vi "Set timebase horizontal scale.vi"(8 "error in (no error)":errorcluster, 9 "Horizontal timebase scale":dbl caption="Timebase horizontal scale", 11 "IVI Refnum in":refnum<k15>) -> (0 "error out":errorcluster, 2 "log string out":string, 3 "IVI Refnum out":refnum<k15>)   [LabVIEW 2017]
uses:
  <instrlib>/Keysight InfiniiVision/Keysight InfiniiVision.lvlib
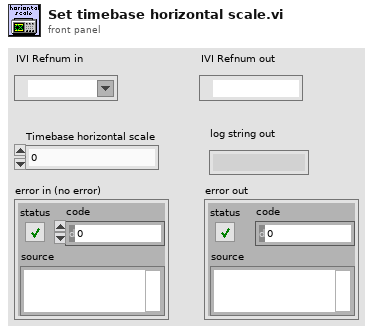
[diagram p1: front panel]
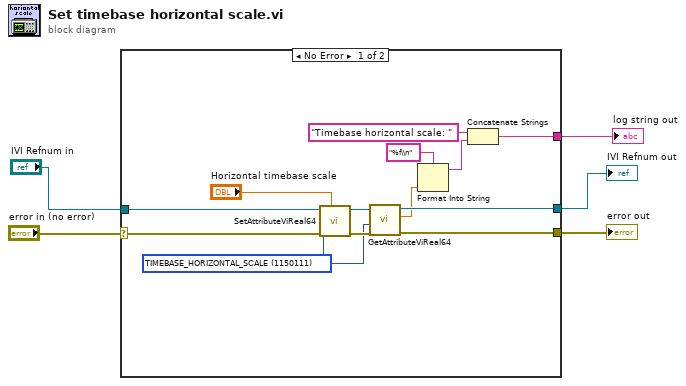
[diagram p0: block diagram]
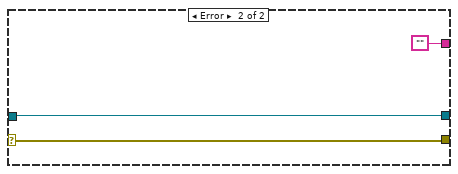
[diagram p2: hidden frame]
diagram:
  n1 = case shown="No Error" "error in (no error)" {
    selector: "error in (no error)" -> [w17 w20]
    tunnel: [w12 w20] -> w5
    tunnel: [w13 w21] -> w4
    tunnel: "IVI Refnum in" -> [w18 w21]
    tunnel: [w7 ""] -> w1
    frame No Error {
      w14 = u32 1150111 items=["ACQUISITION_START_TIME"=1250109, "CHANNEL_PROBE_SKEW"=1150030, "CHANNEL_SCALE"=1150032, "EXTERNAL_PROBE_ATTENUATION"=1150012, "EXTERNAL_RANGE"=1150015, "EXTERNAL_THRESHOLD"=1150680, "EXTERNAL_VERTICAL_POSITION"=1150681, "GLITCH_WIDTH"=1250401, "HORZ_TIME_PER_RECORD"=1250007, "INPUT_IMPEDANCE"=1250103, "INTEGRATE_INPUT_OFFSET"=1150360, "MAX_INPUT_FREQUENCY"=1250006, "MEAS_HIGH_REF"=1250607, "MEAS_LOW_REF"=1250608, "MEAS_MID_REF"=1250609, "PROBE_ATTENUATION"=1250004, "RUNT_HIGH_THRESHOLD"=1250301, "RUNT_LOW_THRESHOLD"=1250302, "TIMEBASE_HORIZONTAL_SCALE"=1150111, "TIMEBASE_WINDOW_HORIZONTAL_SCALE"=1150115, "TIMEBASE_WINDOW_POSITION"=1150113, "TIMEBASE_WINDOW_RANGE"=1150114, "TRIGGER_DELAY_TIME"=1150265, "TRIGGER_EDGE_BURST_IDLE_TIME"=1150248, "TRIGGER_GLITCH_LEVEL"=1150134, "TRIGGER_HOLDOFF"=1250016, "TRIGGER_HOLDOFF_RANDOM_TIME_MAX"=1150683, "TRIGGER_HOLDOFF_RANDOM_TIME_MIN"=1150684, "TRIGGER_LEVEL"=1250017, "TRIGGER_PATTERN_MAX_DURATION"=1150166, "TRIGGER_PATTERN_MIN_WIDTH"=1150158, "TRIGGER_RUNT_QUALIFIER_TIME"=1150191, "TRIGGER_SETUP_AND_HOLD_HOLD_TIME"=1150251, "TRIGGER_SETUP_AND_HOLD_SETUP_TIME"=1150252, "TRIGGER_TRANSITION_QUALIFIER_TIME"=1150257, "TRIGGER_TRANSITION_THRESHOLD_HIGH"=1150428, "TRIGGER_TRANSITION_THRESHOLD_LOW"=1150429, "TRIGGER_WIDTH_THRESHOLD_HIGH"=1150198, "TRIGGER_WIDTH_THRESHOLD_LOW"=1150199, "VERTICAL_OFFSET"=1250002, "VERTICAL_RANGE"=1250001, "WIDTH_HIGH_THRESHOLD"=1250502, "WIDTH_LOW_THRESHOLD"=1250501] ("AttributeID")
      n2 = call <instrlib>:"SetAttributeViReal64.vi"("AttributeValue"="Horizontal timebase scale", "error in (no error)"=w17, "AttributeID"=w14, "instrument handle"=w18) -> ("error out"=w16:errorcluster, "instrument handle out"=w15:refnum<k15>)  [unwired: 6 in]
      n3 = call <instrlib>:"GetAttributeViReal64.vi"("error in (no error)"=w16, "AttributeID"=w14, "instrument handle"=w15) -> ("error out"=w12:errorcluster, "AttributeValue"=w10:dbl, "instrument handle out"=w13:refnum<k15>)  [unwired: 6 in]
      n4 = Format Into String(format string="%f\\n", w10) -> (resulting string=w9:string)  [unwired: 2 in, 1 out]
      n5 = Concatenate Strings("Timebase horizontal scale: " ("string"), w9) -> (w7:string)
    }
    frame Error {
    }
  }
  "error out" <- w5
  "IVI Refnum out" <- w4
  "log string out" <- w1
